vi "Update HTML File.vi"(10 "Plot Data":T1, 11 "Path":path) -> (3 "URL out":string)   [LabVIEW 2020, in "Donut Chart.xctl"]
uses:
  Donut Chart.xctl
  Data Donut Chart.ctl
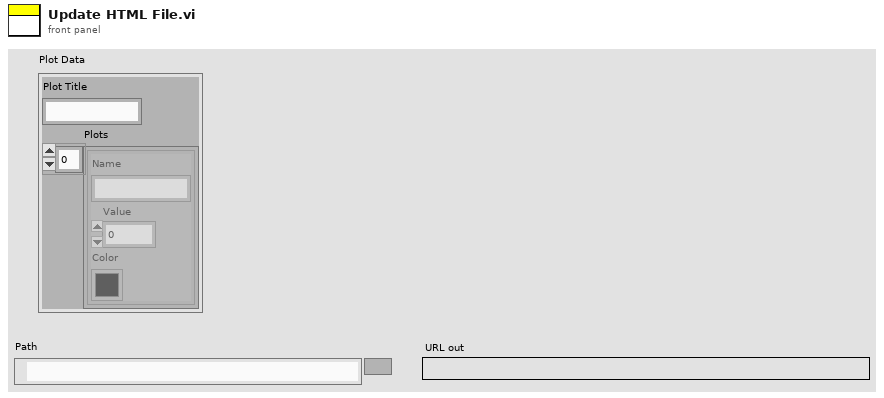
[diagram p1: front panel]
types:
  T1 = typedef "Donut Chart.xctl/Data Donut Chart.ctl" = cluster{"Plot Title":string, "Plots":cluster{"Name":string, "Value":dbl, "Color":u32}[]}
  T2 = enum16{"open", "replace", "create", "open or create", "replace or create", "replace or create with confirmation"}
  T3 = cluster{"Name":string, "Value":dbl, "Color":u32}[]
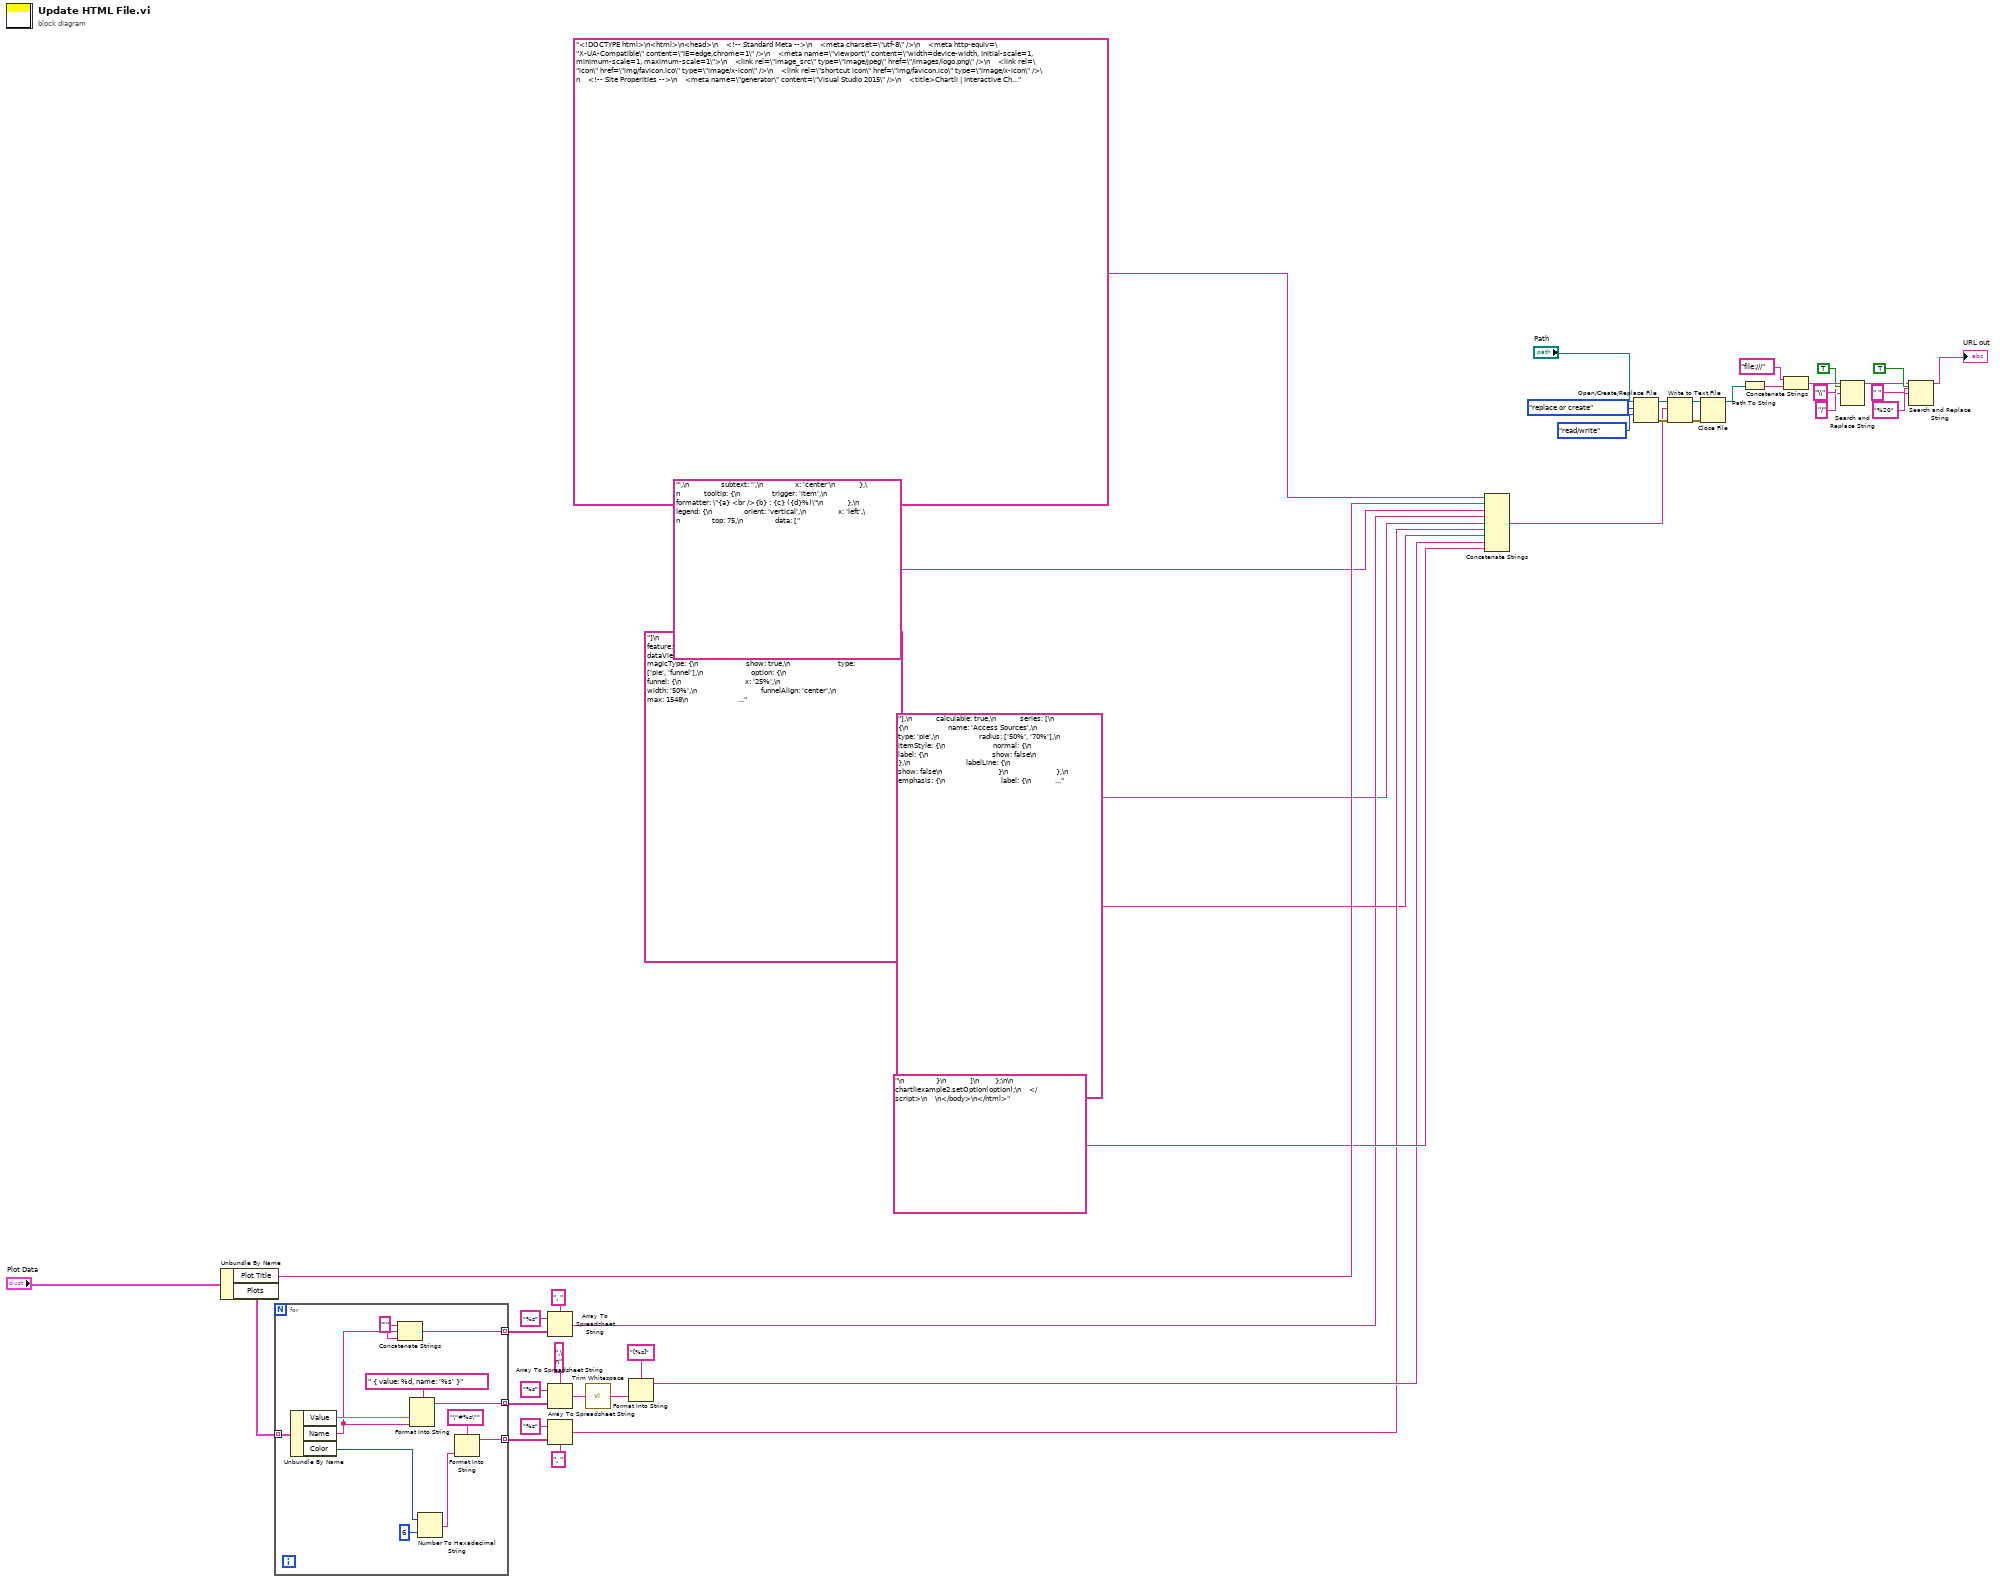
[diagram p0: block diagram]
diagram:
  n1 = Unbundle By Name("Plot Data") -> ("Plot Title"=w43:string, "Plots"=w39:T3)
  n2 = for {
    tunnel: w39 -> [w55] mode=indexing
    tunnel: [w52] -> w35 mode=indexing
    tunnel: [w50] -> w13 mode=indexing
    tunnel: [w47] -> w6 mode=indexing
    w48 = "'" ("string")
    n3 = Unbundle By Name(w55) -> ("Value"=w53:dbl, "Name"=w49:string, "Color"=w44:u32)
    n4 = Concatenate Strings(w48, w49, w48) -> (w47:string)
    n5 = Format Into String(format string=" { value: %d, name: '%s' }", w53, w49) -> (resulting string=w52:string)  [unwired: 2 in, 1 out]
    n6 = Number To Hexadecimal String(1:i16 6 ("width (-)"), 2:w44) -> (0:w45:string)
    n7 = Format Into String(format string="\"#%s\"", w45) -> (resulting string=w50:string)  [unwired: 2 in, 1 out]
  }
  n8 = Array To Spreadsheet String(delimiter (Tab)=", ", array=w6, 3:"%s" ("format string")) -> (spreadsheet string=w5:string)
  n9 = Array To Spreadsheet String(delimiter (Tab)=",\n", array=w35, 3:"%s" ("format string")) -> (spreadsheet string=w37:string)
  n10 = Array To Spreadsheet String(delimiter (Tab)=", ", array=w13, 3:"%s" ("format string")) -> (spreadsheet string=w10:string)
  n11 = call <vilib>:"Trim Whitespace.vi"("string"=w37) -> ("trimmed string"=w36:string)  [unwired: 1 in]
  n12 = Format Into String(format string="[%s]", w36) -> (resulting string=w11:string)  [unwired: 2 in, 1 out]
  n13 = Concatenate Strings("<!DOCTYPE html>\n<html>\n<head>\n    <!-- Standard Meta -->\n    <meta charset=\"utf-8\" />\n    <meta http-equiv=\"X-UA-Compatible\" content=\"IE=edge,chrome=1\" />\n    <meta name=\"viewport\" content=\"width=device-width, initial-scale=1, minimum-scale=1, maximum-scale=1\">\n    <link rel=\"image_src\" type=\"image/jpeg\" href=\"/images/logo.png\" />\n    <link rel=\"icon\" href=\"img/favicon.ico\" type=\"image/x-icon\" />\n    <link rel=\"shortcut icon\" href=\"img/favicon.ico\" type=\"image/x-icon\" />\n    <!-- Site Properities -->\n    <meta name=\"generator\" content=\"Visual Studio 2015\" />\n    <title>Chartli | Interactive Chart</title>\n    <meta name=\"description\" content=\"Chartli Interactive Chart\" />\n    <meta name=\"keywords\" content=\"html5,chart,ui, library, framework, javascript,jquery,graphic,interactive\" />\n    <link href=\"css/semantic.css\" rel=\"stylesheet\" />\n    <link href=\"css/demo.css\" rel=\"stylesheet\" />\n</head>\n\n<body>\n\n    <div id=\"pieChart2\" style=\"height:100%;\"></div>\n\n\n    <script src=\"js/jquery-2.1.4.min.js\"></script>\n    <script src=\"js/chartli.js\"></script>\n        <script type=\"text/javascript\">\n\n        var chartliexample2 = echarts.init(document.getElementById('pieChart2'));\n\n        option = {\n            backgroundColor: '#fffff',\n            title: {\n                text: '", w43, "',\n                subtext: '',\n                x: 'center'\n            },\n            tooltip: {\n                trigger: 'item',\n                formatter: \"{a} <br />{b} : {c} ({d}%)\"\n            },\n            legend: {\n                orient: 'vertical',\n                x: 'left',\n                top: 75,\n                data: [", w5, "]\n            },\n            toolbox: {\n                show: true,\n                feature: {\n                    mark: { show: true },\n                    dataView: { show: true, readOnly: false },\n                    magicType: {\n                        show: true,\n                        type: ['pie', 'funnel'],\n                        option: {\n                            funnel: {\n                                x: '25%',\n                                width: '50%',\n                                funnelAlign: 'center',\n                                max: 1548\n                            }\n                        }\n                    },\n                    restore: { show: true },\n                    saveAsImage: { show: true }\n                }\n            },\n            color: [", w10, "],\n            calculable: true,\n            series: [\n                {\n                    name: 'Access Sources',\n                    type: 'pie',\n                    radius: ['50%', '70%'],\n                    itemStyle: {\n                        normal: {\n                            label: {\n                                show: false\n                            },\n                            labelLine: {\n                                show: false\n                            }\n                        },\n                        emphasis: {\n                            label: {\n                                show: true,\n                                position: 'center',\n                                textStyle: {\n                                    fontSize: '15',\n                                    fontWeight: 'bold'\n                                }\n                            }\n                        }\n                    },\n                    data: ", w11, "\n                }\n            ]\n        };\n\n        chartliexample2.setOption(option);\n    </script>\n    \n</body>\n</html>") -> (w15:string)
  n14 = Open/Create/Replace File(file path (use dialog)="Path", operation (0:open)=T2."replace or create", access (0:read/write)=enum16{"read/write", "read-only", "write-only"}."read/write") -> (refnum out=w31:refnum<file>, error out=w25:errorcluster)  [unwired: 3 in, 1 out]
  n15 = Write to Text File(file (use dialog)=w31, text=w15, error in=w25) -> (refnum out=w29:refnum<file>, error out=w24:errorcluster)  [unwired: 1 in, 1 out]
  n16 = Close File(refnum=w29, error in=w24) -> (path=w26:path)  [unwired: 1 out]
  n17 = Path To String(path=w26) -> (string=w28:string)
  n18 = Concatenate Strings("file:///" ("string"), w28) -> (w23:string)
  n19 = Search and Replace String(replace all?=TRUE ("replace all? (F)"), input string=w23, search string="\\", replace string="/" ("replace string (\"\")")) -> (result string=w16:string)  [unwired: 4 in, 3 out]
  n20 = Search and Replace String(replace all?=TRUE ("replace all? (F)"), input string=w16, search string=" ", replace string="%20" ("replace string (\"\")")) -> (result string=→"URL out":string)  [unwired: 4 in, 3 out]
